vi "Timer.vi"() -> ()   [LabVIEW 2015]
panel:
  in  "Time Target (s)":dbl=2.55 format="%#_13g"
  in  "exit":bool
  in  "Reset":bool
  out "Time has Elapsed":bool
  out "Elapsed Time (s)":dbl
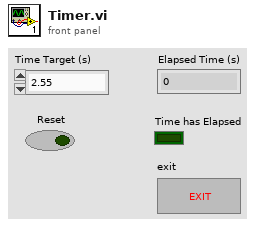
[diagram p1: front panel]
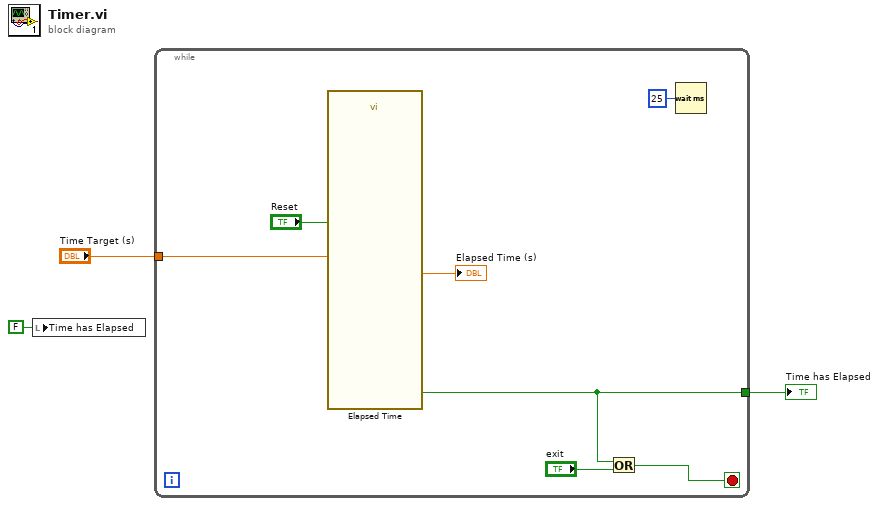
[diagram p0: block diagram]
diagram:
  n1 = local write "Time has Elapsed"(FALSE ("Time has Elapsed")) -> ()
  n2 = while {
    tunnel: [w5] -> w3
    tunnel: "Time Target (s)" -> [w4]
    stop <- w8 stop-if-true
    n3 = call "Elapsed Time"("Time Target (s)"=w4, "Reset"="Reset") -> ("Elapsed Time (s)"=→"Elapsed Time (s)":dbl, "Time has Elapsed"=w5:bool)  [unwired: 10 in, 6 out]
    n4 = Or(x=w5, y="exit") -> (x .or. y?=w8:bool)
    n5 = Wait (ms)(milliseconds to wait=u32 25) -> ()  [unwired: 1 out]
  }
  "Time has Elapsed" <- w3
